vi "overlap_pulses.vi"(9 "stop_read":u32[][](array[numeric]), 10 "start_read":u32[][](array[numeric]), 11 "detections":u32[](array[numeric])) -> (3 "pulses":u32[][](array[numeric]))   [LabVIEW 2018]
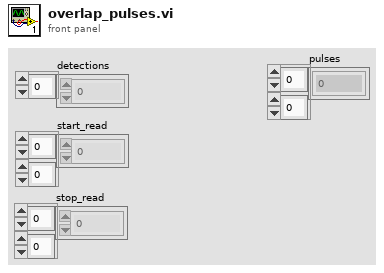
[diagram p1: front panel]
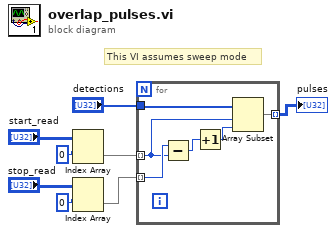
[diagram p0: block diagram]
diagram:
  # "This VI assumes sweep mode"
  n1 = Index Array(array="start_read", index (row)=0) -> (element=w4:u32[])  [unwired: 1 in]
  n2 = Index Array(array="stop_read", index (row)=0) -> (element=w3:u32[])  [unwired: 1 in]
  n3 = for {
    tunnel: w4 -> [w11] mode=indexing
    tunnel: w3 -> [w12] mode=indexing
    tunnel: "detections" -> [w14]
    tunnel: [w13] -> w1 mode=indexing
    n4 = Subtract(x=w12, y=w11) -> (x-y=w10:u32)
    n5 = Increment(x=w10) -> (x+1=w9:u32)
    n6 = Array Subset(array=w14, index=w11, length=w9) -> (w13:u32[])
  }
  "pulses" <- w1
